vi "Rec Save Recordset To File (CR).vi"(5 "overwrite? (F)":bool, 6 "error in (no error)":errorcluster, 7 "save format (XML)":T1=enum."XML", 8 "file name":path, 9 "command-recordset reference":T2) -> (0 "error out":errorcluster, 3 "command-recordset reference out":T2)   [LabVIEW 2020, in "NI_Database_API.lvlib"]
doc: "Saves the recordset identified by the <B>recordset reference</B> to either an XML or ADTG file. The ADTG file format is a proprietary format that only the LabVIEW Database Connectivity Toolkit can interpret. The ADTG format results in a smaller file than the XML format. You can reload both formats into LabVIEW using the DB Tools Load Recordset From File VI.\n\nWire data to the reference input to determine the polymorphic instance to use or manually select the instance."
uses:
  <vilib>/addons/database/NI_Database_API.lvlib
  <vilib>/addons/database/Command-Recordset.llb/Cmd-Rec Object Reference.ctl
  <vilib>/addons/database/Recordset.llb/Rec Save Format.ctl
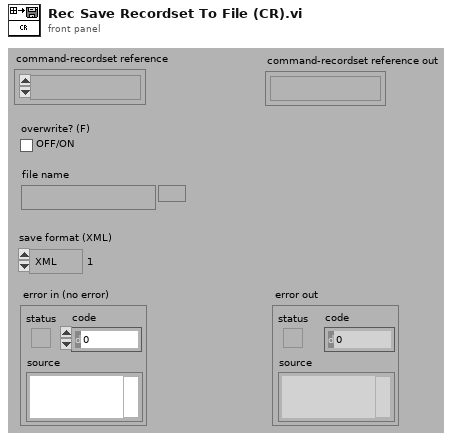
[diagram p1: front panel]
types:
  T1 = typedef "NI_Database_API.lvlib/Rec Save Format.ctl" = enum16{"ADTG", "XML"}
  T2 = typedef "NI_Database_API.lvlib/Cmd-Rec Object Reference.ctl" = refnum<k1>
  T3 = typedef "NI_Database_API.lvlib/Cmd-Rec Data Members.ctl" = cluster{"recordset reference":T4, "command reference":T5}
  T4 = typedef "NI_Database_API.lvlib/Rec ObjectReference.ctl" = refnum<k1>
  T5 = typedef "NI_Database_API.lvlib/Cmd ObjectReference.ctl" = refnum<k1>
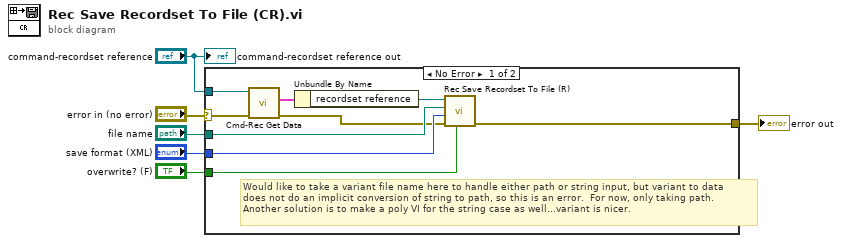
[diagram p0: block diagram]
diagram:
  n1 = case shown="No Error" "error in (no error)" {
    selector: "error in (no error)" -> [w7 w16]
    tunnel: "file name" -> [w15 _]
    tunnel: "overwrite? (F)" -> [w14 _]
    tunnel: [w13 w16] -> w4
    tunnel: "save format (XML)" -> [w12 _]
    tunnel: "command-recordset reference" -> [w8 _]
    frame No Error {
      # "Would like to take a variant file name here to handle either path or string input, but variant to data\ndoes not do an implicit conversion of string to path, so this is an error.  For now, only taking path.\nAnother solution is to make a poly VI for the string case as well...variant is nicer."
      n2 = call <vilib>:"Cmd-Rec Get Data.vi"("error in (no error)"=w7, "command-recordset reference"=w8) -> ("error out"=w9:errorcluster, "data"=w10:T3)  [unwired: 2 in, 2 out]
      n3 = Unbundle By Name(w10) -> ("recordset reference"=w11:T4)
      n4 = call <vilib>:"Rec Save Recordset To File (R).vi"("overwrite? (F)"=w14, "error in (no error)"=w9, "save format (XML)"=w12, "file name"=w15, "recordset reference"=w11) -> ("error out"=w13:errorcluster)  [unwired: 3 in, 1 out]
    }
    frame Error {
    }
  }
  "error out" <- w4
  "command-recordset reference out" <- "command-recordset reference"
